vi "Read Value.vi"(8 "error in (no error)":errorcluster, 11 "int32 in":refnum<class "uint64.lvclass">) -> (0 "error out":errorcluster, 2 "Value":u64, 3 "int32 out":refnum<class "uint64.lvclass">)   [LabVIEW 2020, in "Protobuf RAW.lvlib" / "uint64.lvclass"]
uses:
  uint64.lvclass
  uint64.lvclass/uint64.ctl
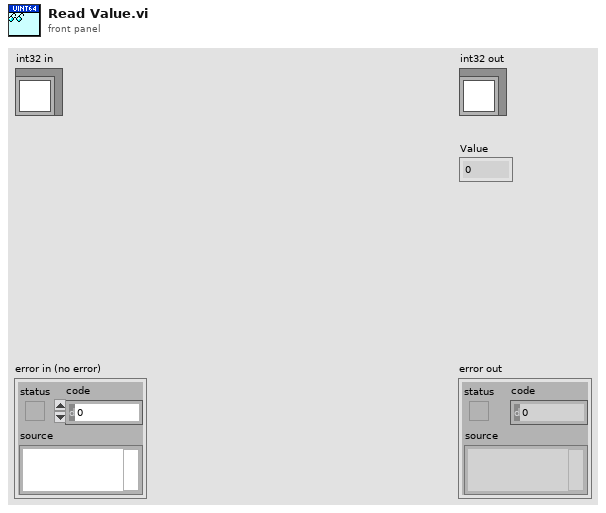
[diagram p1: front panel]
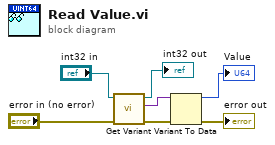
[diagram p0: block diagram]
diagram:
  n1 = call-dynamic "Get Variant.vi"("error in (no error)"="error in (no error)", "Proto Type Common in"="int32 in") -> ("error out"=w6:errorcluster, "Value"=w2:variant, "Proto Type Common out"=→"int32 out":refnum<class "uint64.lvclass">)  [unwired: 7 in]
  n2 = Variant To Data(error in=w6, Variant=w2) -> (data=→"Value":u64, error out=→"error out":errorcluster)  [unwired: 1 in]
